vi "Port D_A Output Mode.vi"(7 "Read Value? (F)":bool, 8 "error in (no error)":errorcluster, 9 "Port Output Mode (Fixed)":T1, 10 "Port (1)":T2=enum."1", 11 "VISA resource name":refnum<visa-resource-name>) -> (0 "error out":errorcluster, 1 "Port Output Mode":T1, 3 "VISA resource name out":refnum<visa-resource-name>)   [LabVIEW 2013, in "SRS SR400.lvlib"]
doc: "<B>PM i { ,j }</B>\n\nThe PM command sets and reads the rear panel PORT1 and PORT2 D/A output modes. i=1 or 2 to select PORT1 or PORT 2 and is required. If j is included, the mode is set to FIXED, j=0, or SCAN, j=1. If j is absent, the mode is returned. The mode may be changed during a scan. If it is changed to SCAN, the level begins scanning from the start value on the next count period. If it is changed to FIXED, the level returns to the start value immediately."
uses:
  <instrlib>/SRS SR400/SRS SR400.lvlib
  <instrlib>/SRS SR400/Public/Typedefs/Port.ctl
  <instrlib>/SRS SR400/Public/Typedefs/Port Output Mode.ctl
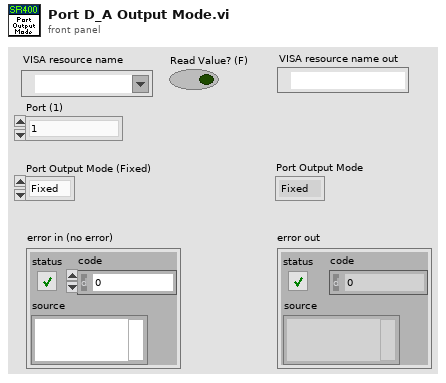
[diagram p1: front panel]
types:
  T1 = typedef "SRS SR400.lvlib/Port Output Mode.ctl" = enum16{"Fixed", "Scan"}
  T2 = typedef "SRS SR400.lvlib/Port.ctl" = enum16{"(not used)", "1", "2"}
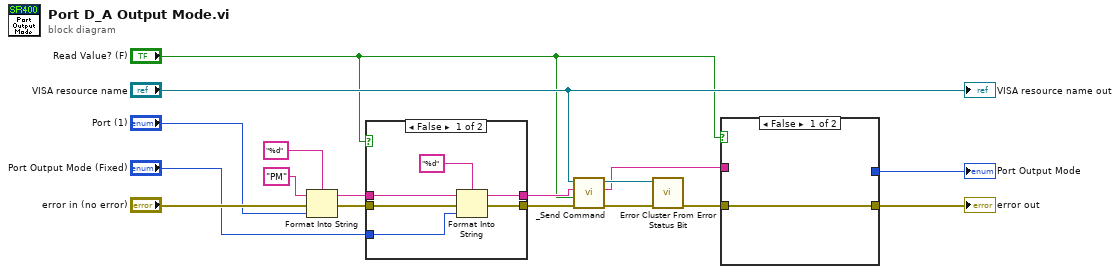
[diagram p0: block diagram]
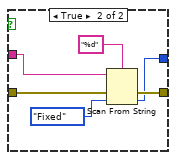
[diagram p2: hidden frame]
diagram:
  n1 = Format Into String(format string="%d", initial string="PM" ("command"), error in="error in (no error)", "Port (1)") -> (resulting string=w15:string, error out=w16:errorcluster)
  n2 = case shown="False" "Read Value? (F)" {
    tunnel: w16 -> [w23 w24]
    tunnel: w15 -> [w18 w25]
    tunnel: [w21 w25] -> w12
    tunnel: [w20 w24] -> w11
    tunnel: "Port Output Mode (Fixed)" -> [w19 _]
    frame False {
      n3 = Format Into String(format string="%d", initial string=w18, error in=w23, w19) -> (resulting string=w21:string, error out=w20:errorcluster)
    }
    frame True {
    }
  }
  n4 = call <instrlib>:"_Send Command.vi"("error in (no error)"=w11, "Read Value? (F)"="Read Value? (F)", "Command"=w12, "VISA resource name"="VISA resource name") -> ("error out"=w7:errorcluster, "Response"=w2:string, "VISA resource name out"=w8:refnum<visa-resource-name>)  [unwired: 5 out]
  n5 = call <instrlib>:"Error Cluster From Error Status Bit.vi"("error in (no error)"=w7, "VISA resource name"=w8) -> ("error out"=w4:errorcluster)  [unwired: 8 in, 1 out]
  n6 = case shown="False" "Read Value? (F)" {
    tunnel: w4 -> [w26 w32]
    tunnel: [w26 w31] -> w3
    tunnel: w2 -> [_ w28]
    tunnel: [_ w27] -> w1
    frame False {
    }
    frame True {
      n7 = Scan From String(format string="%d", input string=w28, error in=w32, default 1=Port_Output_Mode."Fixed" ("Port Output Mode (Fixed)")) -> (error out=w31:errorcluster, output 1=w27:T1)  [unwired: 1 in, 2 out]
    }
  }
  "error out" <- w3
  "Port Output Mode" <- w1
  "VISA resource name out" <- "VISA resource name"
